vi "JSON to Cluster.vi"() -> ()   [LabVIEW 2014]
panel:
  in  "error in":errorcluster
  in  "JSON String":string="{\n    \"firstName\": \"John\",\n    \"lastName\": \"Smith\",\n    \"age\": 25,\n    \"address\": {\n        \"streetAddress\": \"21 2nd Street\",\n        \"city\": \"New York\",\n        \"state\": \"NY\",\n        \"postalCode\": 10021\n    },\n    \"phoneNumbers\": [\n        {\n            \"type\": \"home\",\n            \"number\": \"212 555-1234\"\n        },\n        {\n            \"type\": \"fax\",\n            \"number\": \"646 555-4567\"\n        }\n    ]\n}"
  # "1. Paste JSON string into control and run VI\n2. New VI is created that contains cluster \nrepresentation of the object, and that can\nbe used with the Unflatten from JSON VI"
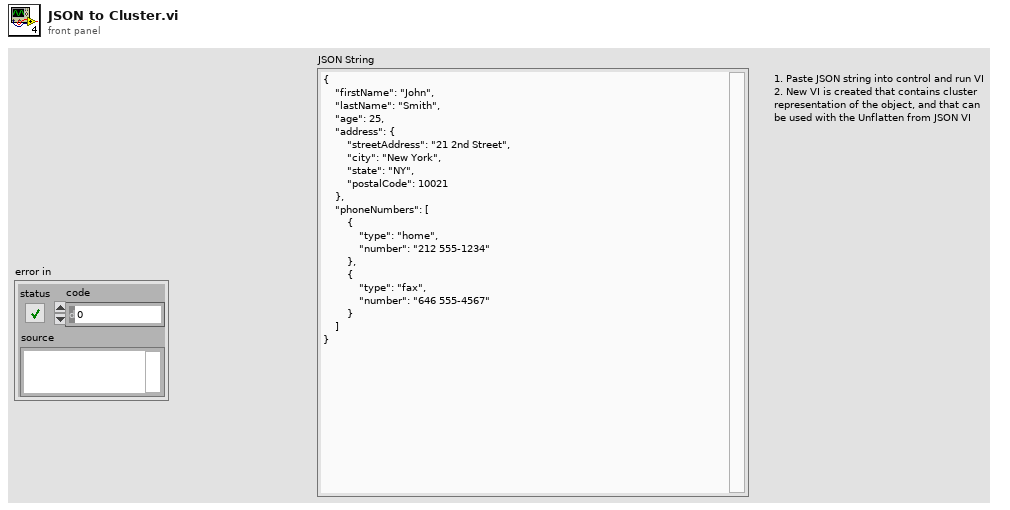
[diagram p1: front panel]
types:
  T1 = typedef "Token.ctl" = enum16{"End", "Boolean", "Named Cluster", "Unnamed Cluster", "Array", "String", "Decimal", "FloatingPoint", "End Array", "End Cluster"}
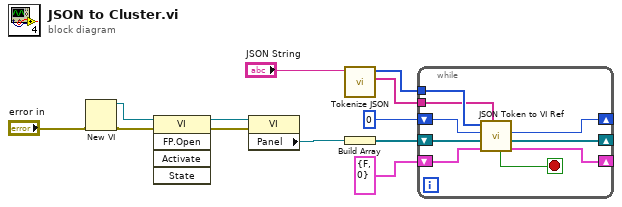
[diagram p0: block diagram]
diagram:
  n1 = New VI(8:"error in") -> (0:w2:errorcluster, 3:w1:refnum<vi>)  [unwired: 6 in]
  n2 = invoke class="VI" method="FP.Open"(reference=w1, error in=w2) -> (reference out=w8:refnum<vi>, error out=w6:errorcluster)  [unwired: 3 in, 3 out]
  n3 = property class="VI"(reference=w8, error in=w6) -> ("Panel"=w7:refnum<vi>)  [unwired: 2 out]
  n4 = call "Tokenize JSON.vi"("JSON String"="JSON String") -> ("Variable Names"=w10:string[], "Token Array"=w11:T1[])  [unwired: 9 in]
  n5 = Build Array(w7) -> (w4:refnum<vi>[])
  n6 = while {
    tunnel: w11 -> [w20]
    tunnel: w10 -> [w19]
    shift-right: [w17] -> _
    shift-left: 0 -> [w18]
    shift-right: [w16] -> _
    shift-left: w4 -> [w21]
    shift-right: [w13] -> _
    shift-left: cluster{"In Array?":bool, "Cluster Level":i32} {"In Array?"=FALSE, "Cluster Level"=0} ("Inception Tracking") -> [w14]
    stop <- w15 stop-if-true
    n7 = call "JSON Token to VI Ref.vi"("Variable Names"=w19, "Inception Tracking"=w14, "Parent Ref"=w21, "index"=w18, "Token Array"=w20) -> ("Inception Tracking Out"=w13:cluster{"In Array?":bool, "Cluster Level":i32}, "Parent Ref Out"=w16:refnum<vi>[], "index out"=w17:i32, "End?"=w15:bool)  [unwired: 3 in]
  }
